vi "S2DS_Read or load config file (SubVI).vi"(5 "False channel (in)":string[][](array[string]), 7 "Loading information in":bool[](array[boolean]), 8 "error in (no error)":errorcluster, 9 "Update present value?":bool, 10 "All channel parameters (in)":T1 {"Scan parameters"."Y data taking" items=["in both direction", "in up direction only", "in down direction only"]; "Scan parameters"."X data taking" items=["in both direction", "in up direction only", "in down direction only"]}, 11 "selected path":path) -> (0 "error out":errorcluster, 1 "False channel (out)":string[][](array[string]), 2 "All channel parameters (out)":T1 {"Scan parameters"."Y data taking" items=["in both direction", "in up direction only", "in down direction only"]; "Scan parameters"."X data taking" items=["in both direction", "in up direction only", "in down direction only"]}, 3 "file path":path)   [LabVIEW 2025]
uses:
  TYPE DEFS/S2DS_All Channel Parameters.ctl
  TYPE DEFS/S2DS_WC info.ctl
  TYPE DEFS/S2DS_Single WC info.ctl
  TYPE DEFS/S2DS_RC info.ctl
  TYPE DEFS/S2DS_Single RC info.ctl
  TYPE DEFS/S2DS_DAC info new.ctl
  TYPE DEFS/S2DS_Single DC info.ctl
  TYPE DEFS/S2DS_Array Inst Info.ctl
  TYPE DEFS/S2DS_Sweep Info.ctl
  <vilib>/Utility/config.llb/Read Key (String).vi
  <vilib>/Utility/config.llb/NI_LVConfig.lvlib
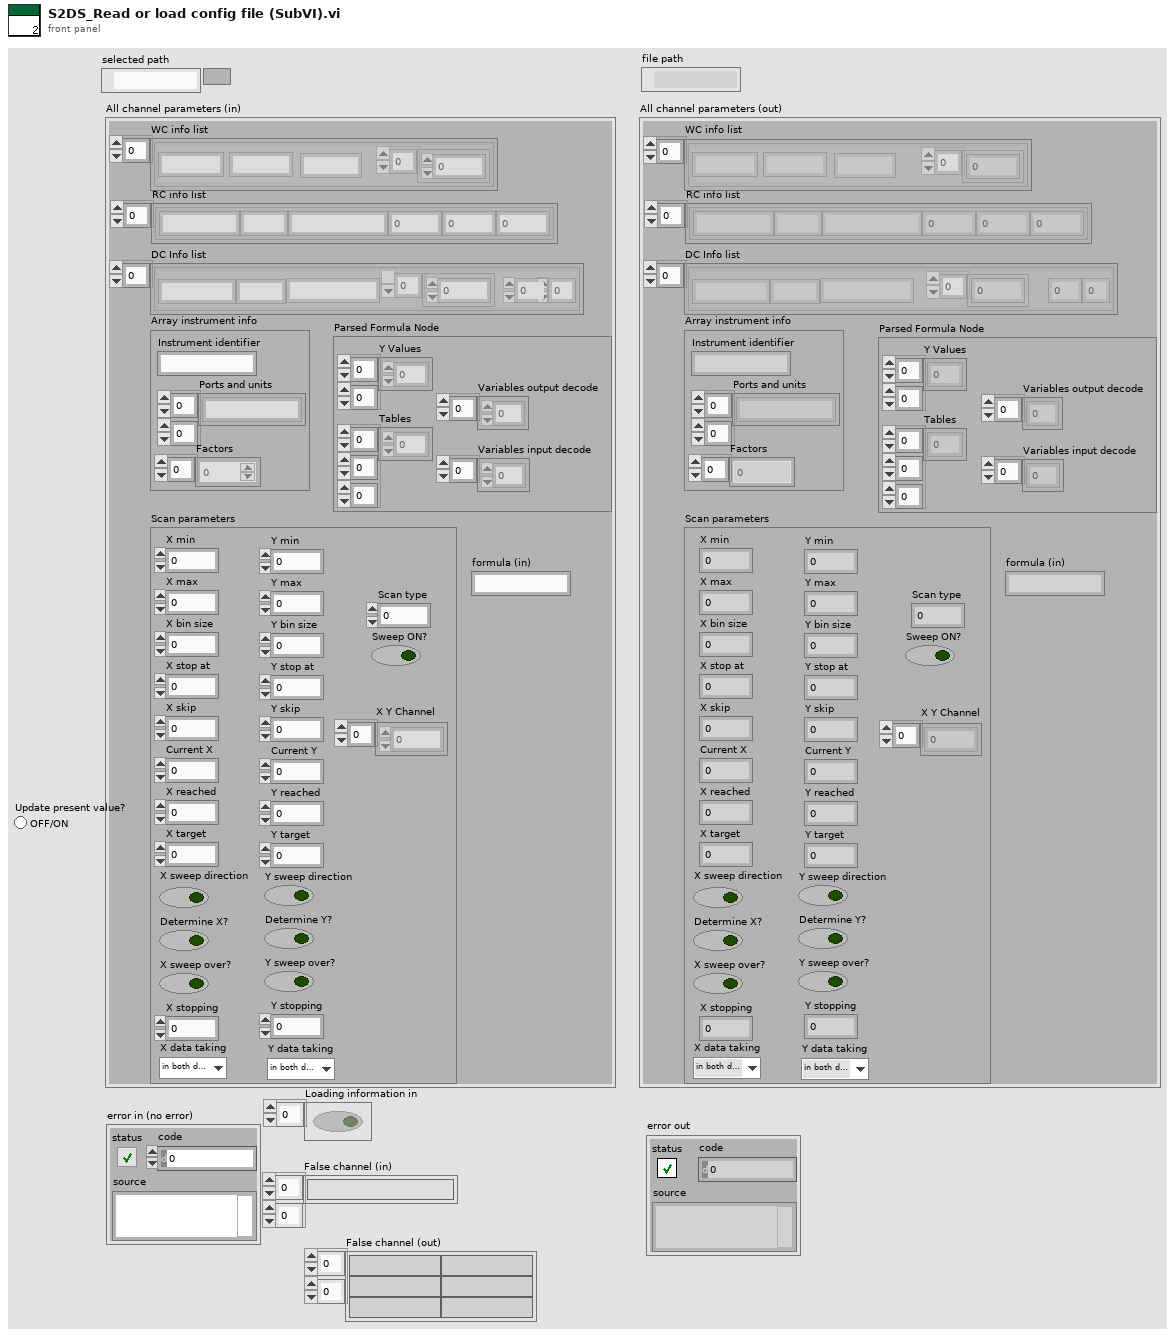
[diagram p1: front panel]
types:
  T1 = typedef "S2DS_All Channel Parameters.ctl" = cluster{"WC info list":T2, "RC info list":T4, "DC Info list":T6, "Array instrument info":T8, "Scan parameters":T9, "Parsed Formula Node":cluster{"Y Values":dbl[][], "Tables":i32[][][], "Variables input decode":i32[], "Variables output decode":i32[]}, "formula (in)":string}
  T2 = typedef "S2DS_WC info.ctl" = T3[]
  T3 = typedef "S2DS_Single WC info.ctl" = cluster{"Instrument identifier":string, "Write channel parameters":dbl[], "Name":string, "Unit":string}
  T4 = typedef "S2DS_RC info.ctl" = T5[]
  T5 = typedef "S2DS_Single RC info.ctl" = cluster{"Instrument identifier":string, "Factor":dbl, "Averaging":i32, "Wait (ms)":i32, "Unit":string, "Name":string}
  T6 = typedef "S2DS_DAC info new.ctl" = T7[]
  T7 = typedef "S2DS_Single DC info.ctl" = cluster{"Operation identifier":string, "DC parameters":dbl[], "U":i32, "V":i32, "Name":string, "Unit":string}
  T8 = typedef "S2DS_Array Inst Info.ctl" = cluster{"Instrument identifier":string, "Ports and units":string[][], "Factors":dbl[]}
  T9 = typedef "S2DS_Sweep Info.ctl" = cluster{"X min":ext, "X max":dbl, "Y min":dbl, "Y max":dbl, "X bin size":dbl, "Y bin size":dbl, "X stop at":dbl, "Y stop at":dbl, "X skip":u64, "Y skip":u64, "Current X":dbl, "Current Y":dbl, "X reached":i32, "Y reached":i32, "X target":dbl, "Y target":dbl, "Sweep ON?":bool, "X sweep direction":bool, "Y sweep direction":bool, "Determine X?":bool, "Determine Y?":bool, "X sweep over?":bool, "Y sweep over?":bool, "Scan type":i32, "X stopping":i32, "Y stopping":i32, "X Y Channel":u16[], "X data taking":u16, "Y data taking":u16}
  T10 = typedef "NI_LVConfig.lvlib/Config Data RefNum.ctl" = refnum<k1>
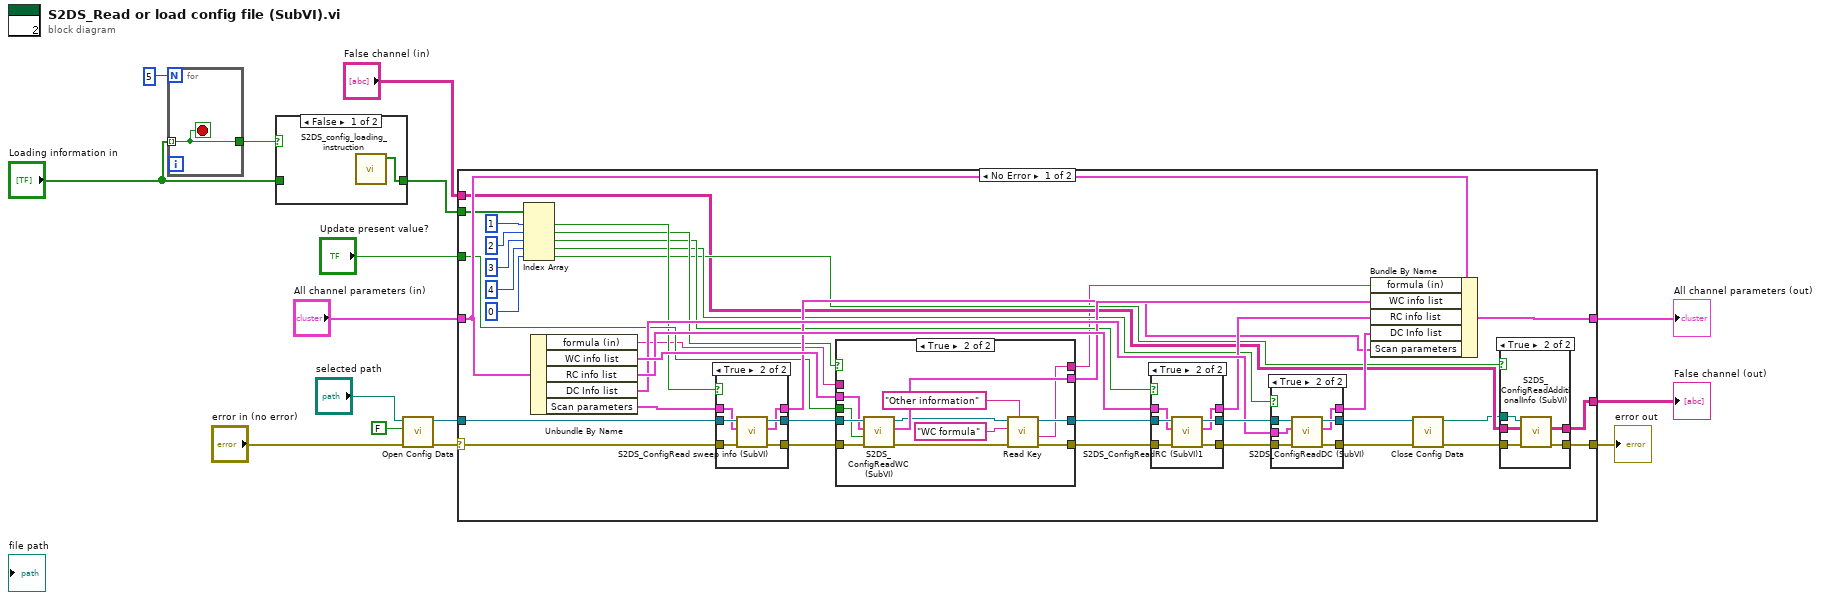
[diagram p0: block diagram]
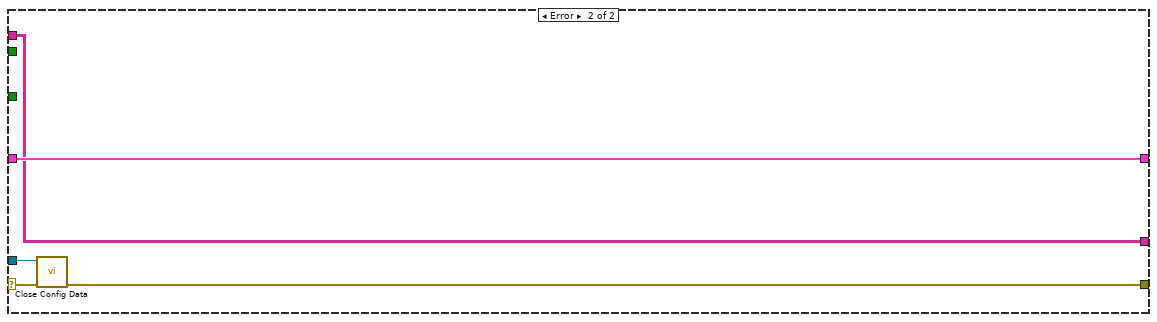
[diagram p8: hidden frame]
diagram:
  n1 = for {
    N: 5 -> [_]
    tunnel: "Loading information in" -> [w16] mode=indexing
    tunnel: [w16] -> w5
    stop <- w16 stop-if-true
  }
  n2 = case shown="False" w5 {
    tunnel: [w17 w18] -> w7
    tunnel: "Loading information in" -> [_ w18]
    frame False {
      n3 = call "S2DS_config_loading_instruction.vi"() -> ("Loading information out"=w17:bool[])  [unwired: 11 in]
    }
    frame True {
    }
  }
  n4 = call <vilib>:"Open Config Data.vi"("error in (no error)"="error in (no error)", "create file if necessary (T)"=FALSE ("create file if necessary? (T)"), "configuration file path"="selected path") -> ("error out"=w11:errorcluster, "refnum"=w12:T10)  [unwired: 6 in, 1 out]
  n5 = case shown="No Error" w11 {
    selector: w11 -> [w50 w109]
    tunnel: w12 -> [w53 w110]
    tunnel: [w25 w108] -> w1
    tunnel: "All channel parameters (in)" -> [w45 w112]
    tunnel: [w40 w112] -> w9
    tunnel: "Update present value?" -> [w39 _]
    tunnel: w7 -> [w38 _]
    tunnel: [w27 w111] -> w3
    tunnel: "False channel (in)" -> [w26 w111]
    frame No Error {
      n6 = Index Array(array=w38, index #1=1 ("index"), index #2=2 ("index"), index #3=3 ("index"), index #4=4 ("index"), index #5=0 ("index")) -> (element #1=w34:bool, element #2=w33:bool, element #3=w32:bool, element #4=w30:bool, element #5=w28:bool)
      n7 = Unbundle By Name(w45) -> ("formula (in)"=w20:string, "WC info list"=w49:T2, "RC info list"=w48:T4, "DC Info list"=w47:T6, "Scan parameters"=w46:T9)
      n8 = case shown="True" w34 {
        tunnel: w53 -> [w99 w107]
        tunnel: [w100 w106] -> w52
        tunnel: [w99 w105] -> w51
        tunnel: w50 -> [w100 w104]
        tunnel: w46 -> [w101 w103]
        tunnel: [w101 w102] -> w41
        frame False {
        }
        frame True {
          n9 = call "S2DS_ConfigRead sweep info (SubVI).vi"("error in (no error)"=w104, "Scan parameters in"=w103, "Refnum in"=w107) -> ("error out"=w106:errorcluster, "Scan information (out)"=w102:T9, "Refnum out"=w105:T10)  [unwired: 6 in]
        }
      }
      n10 = case shown="True" w33 {
        tunnel: [w84 w90] -> w55
        tunnel: [w86 w92] -> w54
        tunnel: w52 -> [w84 w98]
        tunnel: w51 -> [w86 w97]
        tunnel: w49 -> [w85 w96]
        tunnel: [w85 w95] -> w44
        tunnel: w39 -> [_ w94]
        tunnel: [w83 w87] -> w19
        tunnel: w20 -> [w83 _]
        frame False {
        }
        frame True {
          n11 = call "S2DS_ConfigReadWC (SubVI).vi"("Refnum in"=w97, "WC Info list (in)"=w96, "Update present value?"=w94, "error in (no error)"=w98) -> ("Refnum out"=w93:T10, "WC Info list (out)"=w95:T2, "error out"=w91:errorcluster)  [unwired: 3 in]
          n12 = call-poly <vilib>:"Read Key.vi"("section"="Other information", "error in (no error)"=w91, "key"="WC formula", "refnum"=w93) -> ("error out"=w90:errorcluster, "value"=w87:string, "refnum out"=w92:T10)  [unwired: 4 in, 1 out]
        }
      }
      n13 = case shown="True" w32 {
        tunnel: [w76 w82] -> w57
        tunnel: [w74 w81] -> w56
        tunnel: w55 -> [w74 w80]
        tunnel: w54 -> [w76 w79]
        tunnel: w48 -> [w75 w78]
        tunnel: [w75 w77] -> w43
        frame False {
        }
        frame True {
          n14 = call "S2DS_ConfigReadRC (SubVI)1.vi"("Refnum in"=w79, "RC Info list (in)"=w78, "error in (no error)"=w80) -> ("Refnum out"=w82:T10, "RC Info list (out)"=w77:T4, "error out"=w81:errorcluster)  [unwired: 4 in]
        }
      }
      n15 = case shown="True" w30 {
        tunnel: w57 -> [w67 w73]
        tunnel: w56 -> [w65 w72]
        tunnel: [w67 w71] -> w24
        tunnel: [w65 w70] -> w23
        tunnel: w47 -> [w66 w69]
        tunnel: [w66 w68] -> w42
        frame False {
        }
        frame True {
          n16 = call "S2DS_ConfigReadDC (SubVI).vi"("Refnum in"=w73, "DC Info list (in)"=w69, "error in (no error)"=w72) -> ("Refnum out"=w71:T10, "DC Info list (out)"=w68:T6, "error out"=w70:errorcluster)  [unwired: 4 in]
        }
      }
      n17 = Bundle By Name(cluster=w45, "formula (in)"=w19, "WC info list"=w44, "RC info list"=w43, "DC Info list"=w42, "Scan parameters"=w41) -> (w40:T1)
      n18 = call <vilib>:"Close Config Data.vi"("error in (no error)"=w23, "refnum"=w24) -> ("error out"=w21:errorcluster, "file path"=w22:path)  [unwired: 8 in]
      n19 = case shown="True" w28 {
        tunnel: [w59 w64] -> w27
        tunnel: w26 -> [w59 w63]
        tunnel: w22 -> [_ w60]
        tunnel: [w58 w62] -> w25
        tunnel: w21 -> [w58 w61]
        frame False {
        }
        frame True {
          n20 = call "S2DS_ConfigReadAdditionalInfo (SubVI).vi"("error in (no error)"=w61, "False channel (in) in"=w63, "file path (use dialog)"=w60) -> ("error out"=w62:errorcluster, "False channel (in) out"=w64:string[][])  [unwired: 7 in]
        }
      }
    }
    frame Error {
      n21 = call <vilib>:"Close Config Data.vi"("error in (no error)"=w109, "refnum"=w110) -> ("error out"=w108:errorcluster)  [unwired: 8 in, 1 out]
    }
  }
  "error out" <- w1
  "All channel parameters (out)" <- w9
  "False channel (out)" <- w3
